vi "Measure IV curves sequence in same file 2420.vi"() -> ()   [LabVIEW 2014]
uses:
  Environmental Chamber LabVIEW and Instruments/Drivers and Software/LabVIEW 8.2 Drivers/keithley_24xx/Keithley 24XX/Public/Data/Read (Single Point).vi
  <vilib>/Utility/file.llb/Write To Spreadsheet File (string).vi
  Environmental Chamber LabVIEW and Instruments/Drivers and Software/keithley_24xx/Keithley 24XX/Keithley 24XX.lvlib
panel:
  in  "voltage settings":T1={"Vi (V)"=-0.5, "Vf (V)"=0.5, "steps"=100.0, "# of curves"=1, "Delay (min)"=0.02} {"Delay (min)" min=0.0 format="%#_13g"; "# of curves" step=1}
  out "File path":path
  in  "STOP":bool
  out "2420 IV curve":cluster{"X":dbl[], "Y":dbl[]}[](graph)
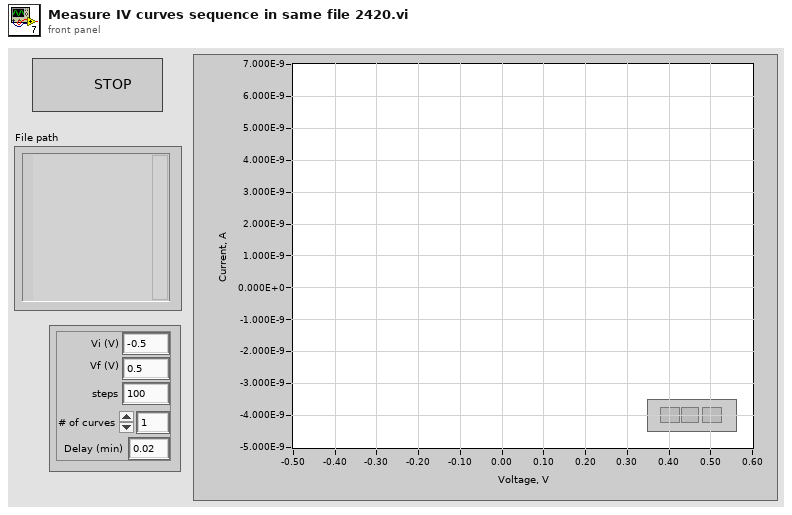
[diagram p1: front panel]
types:
  T1 = cluster{"Vi (V)":dbl, "Vf (V)":dbl, "steps":dbl, "# of curves":u32, "Delay (min)":dbl}
  T2 = enum16{"open", "open or create", "create or replace", "create", "open (read only)"}
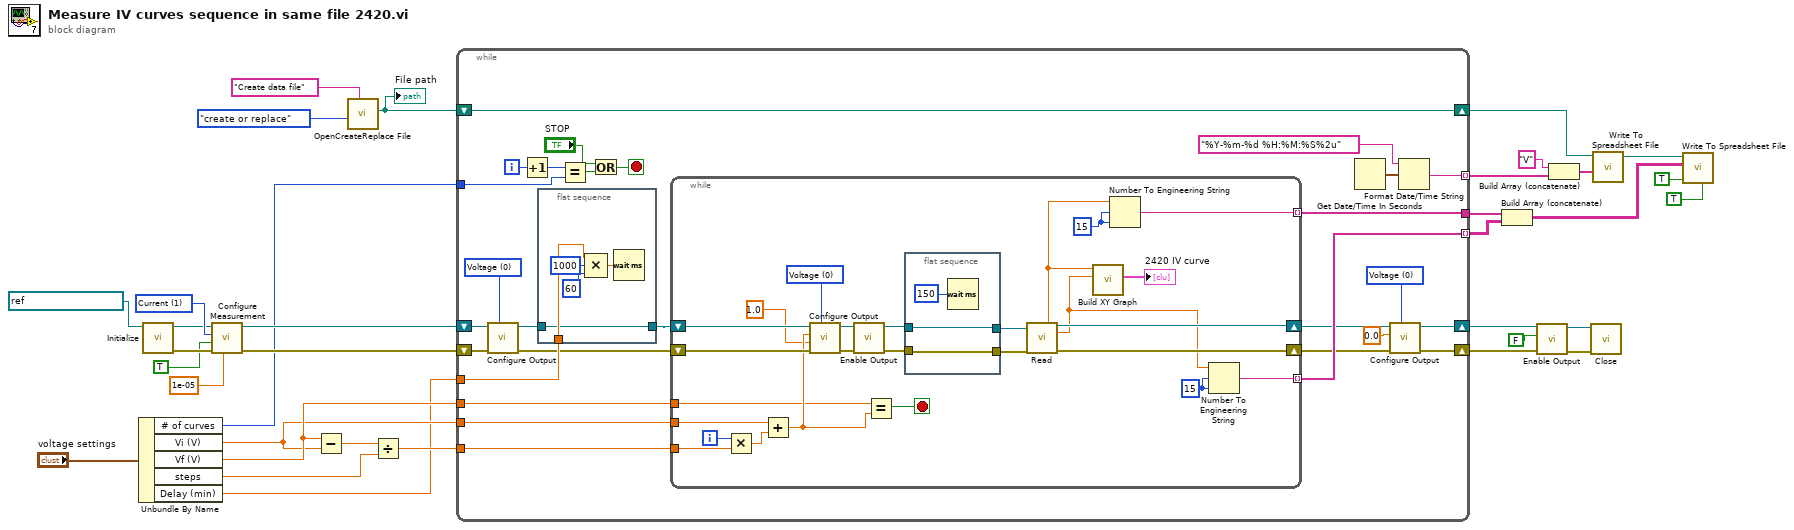
[diagram p0: block diagram]
diagram:
  w26 = u16 1 items=["Volts", "Current", "Resistance"] ("Function (0: Volts)")
  n1 = Unbundle By Name("voltage settings") -> ("# of curves"=w15:u32, "Vi (V)"=w16:dbl, "Vf (V)"=w17:dbl, "steps"=w18:dbl, "Delay (min)"=w14:dbl)
  n2 = call "Initialize.vi"("VISA resource name"=refnum<visa-resource-name> "GPIB1::24::INSTR") -> ("error out"=w22:errorcluster, "VISA resource name out"=w23:refnum<visa-resource-name>)  [unwired: 9 in]
  n3 = call "Configure Measurement.vi"("Manual Range (1.0)"=1e-05, "error in (no error)"=w22, "Enable Auto Range (T:Enable)"=TRUE, "Function (0: Volts)"=w26, "VISA resource name"=w23) -> ("error out"=w25:errorcluster, "VISA resource name out"=w24:refnum<visa-resource-name>)  [unwired: 5 in]
  n4 = Subtract(x=w17, y=w16) -> (x-y=w34:dbl)
  n5 = call "OpenCreateReplace File.vi"("prompt"="Create data file", "function (open:0)"=T2."create or replace") -> ("new file path"=w11:path)  [unwired: 6 in, 3 out]
  "File path" <- w11
  n6 = Divide(x=w34, y=w18) -> (x/y=w33:dbl)
  n7 = while {
    tunnel: w17 -> [w62]
    tunnel: w16 -> [w61]
    tunnel: w33 -> [w60]
    shift-right: [w42] -> w28
    shift-left: w25 -> [w36]
    shift-right: [w44] -> w29
    shift-left: w24 -> [w38]
    shift-right: [w53] -> w9
    shift-left: w11 -> [w53]
    tunnel: w15 -> [w55]
    tunnel: w14 -> [w54]
    tunnel: [w50] -> w6 mode=indexing
    tunnel: [w49] -> w4
    tunnel: [w48] -> w3 mode=indexing
    i -> [w47]
    stop <- w59 stop-if-true
    w39 = u16 0 items=["Voltage", "Current"] ("Source Mode  (0: Voltage)")
    w46 = u16 0 items=["Voltage", "Current"] ("Source Mode  (0: Voltage)")
    n8 = call "Configure Output.vi"("Source Mode  (0: Voltage)"=w39, "error in (no error)"=w36, "VISA resource name"=w38) -> ("error out"=w35:errorcluster, "VISA resource name out"=w37:refnum<visa-resource-name>)  [unwired: 7 in]
    n9 = Increment(x=w47) -> (x+1=w57:i32)
    n10 = flat-sequence {
      tunnel: w37 -> [w63]
      tunnel: w54 -> [w64]
      tunnel: [w63] -> w40
      frame #0 {
        n11 = Compound Arithmetic op=MULTIPLY(w64, u32 1000 ("value"), u32 60 ("value")) -> (w67:dbl)
        n12 = Wait (ms)(milliseconds to wait=w67) -> ()  [unwired: 1 out]
      }
    }
    n13 = Equal?(x=w57, y=w55) -> (x = y?=w56:bool)
    n14 = Or(x="STOP", y=w56) -> (x .or. y?=w59:bool)
    n15 = while {
      tunnel: [w86] -> w48 mode=indexing
      shift-right: [w92] -> w43
      shift-left: w35 -> [w91]
      shift-right: [w93] -> w45
      shift-left: w40 -> [w90]
      tunnel: w60 -> [w69]
      tunnel: w61 -> [w81]
      tunnel: [w80] -> w49 mode=indexing
      tunnel: w62 -> [w71]
      i -> [w70]
      stop <- w73 stop-if-true
      w77 = i16 15 ("precision (6)")
      w78 = i16 15 ("precision (6)")
      w87 = u16 0 items=["Voltage", "Current"] ("Source Mode  (0: Voltage)")
      n16 = Multiply(x=w70, y=w69) -> (x*y=w79:dbl)
      n17 = Add(x=w81, y=w79) -> (x+y=w72:dbl)
      n18 = call "Configure Output.vi"("Source Mode  (0: Voltage)"=w87, "error in (no error)"=w91, "Compliance  Level (0.1)"=1.0, "Output Level (0)"=w72, "VISA resource name"=w90) -> ("error out"=w89:errorcluster, "VISA resource name out"=w88:refnum<visa-resource-name>)  [unwired: 5 in]
      n19 = call "Enable Output.vi"("error in (no error)"=w89, "VISA resource name"=w88) -> ("error out"=w82:errorcluster, "VISA resource name out"=w85:refnum<visa-resource-name>)  [unwired: 8 in]
      n20 = Equal?(x=w71, y=w72) -> (x = y?=w73:bool)
      n21 = flat-sequence {
        tunnel: [w96] -> w84
        tunnel: w85 -> [w96]
        tunnel: w82 -> [w95]
        tunnel: [w95] -> w83
        frame #0 {
          n22 = Wait (ms)(milliseconds to wait=150 ("x")) -> ()  [unwired: 1 out]
        }
      }
      n23 = call-poly "Read.vi"("VISA resource name"=w84, "error in (no error)"=w83) -> ("Voltage"=w75:sgl, "VISA resource name out"=w93:refnum<visa-resource-name>, "Current"=w76:sgl, "error out"=w92:errorcluster)  [unwired: 7 in, 3 out]
      n24 = call "Build XY Graph"("Y Input"=w76, "X Input"=w75) -> ("XY Graph"=→"2420 IV curve":cluster{"X":dbl[], "Y":dbl[]}[])  [unwired: 8 in, 1 out]
      n25 = Number To Engineering String(2:w77, 3:w77, 4:w75) -> (0:w80:string)  [unwired: 1 in]
      n26 = Number To Engineering String(2:w78, 3:w78, 4:w76) -> (0:w86:string)  [unwired: 1 in]
    }
    n27 = Get Date/Time In Seconds() -> (seconds since 1Jan1904=w52:timestamp)
    n28 = call "Configure Output.vi"("Source Mode  (0: Voltage)"=w46, "error in (no error)"=w43, "Output Level (0)"=0.0, "VISA resource name"=w45) -> ("error out"=w42:errorcluster, "VISA resource name out"=w44:refnum<visa-resource-name>)  [unwired: 6 in]
    n29 = Format Date/Time String(time format string (%c)="%Y-%m-%d %H:%M:%S%2u", seconds (now)=w52) -> (date/time string=w50:string)  [unwired: 1 in]
  }
  n30 = Build Array (concatenate)(w4, w3) -> (w2:string[][])
  n31 = call "Enable Output.vi"("error in (no error)"=w28, "Enable Output (T: Enable)"=FALSE, "VISA resource name"=w29) -> ("error out"=w30:errorcluster, "VISA resource name out"=w32:refnum<visa-resource-name>)  [unwired: 7 in]
  n32 = Build Array (concatenate)("V", w6) -> (w5:string[])
  n33 = call "Close.vi"("error in (no error)"=w30, "VISA resource name"=w32) -> ()  [unwired: 9 in, 1 out]
  n34 = call-poly <vilib>:"Write To Spreadsheet File.vi"("1D data"=w5, "file path (dialog if empty)"=w9) -> ("new file path (Not A Path if cancelled)"=w8:path)  [unwired: 6 in]
  n35 = call-poly <vilib>:"Write To Spreadsheet File.vi"("transpose? (no:F)"=TRUE, "append to file? (new file:F)"=TRUE ("transpose? (no:F)"), "2D data"=w2, "file path (dialog if empty)"=w8) -> ()  [unwired: 4 in, 1 out]
